vi "ScaleWaveData.vi"(8 "error in (no error)":errorcluster, 11 "dDataIn":dbl[](array[numeric])) -> (0 "error out":errorcluster, 3 "dDataOut":dbl[](array[numeric]))   [LabVIEW 2014, in "FGenPlugins.lvlib" / "NiPxi6733.lvclass"]
uses:
  NiPxi6733.lvclass
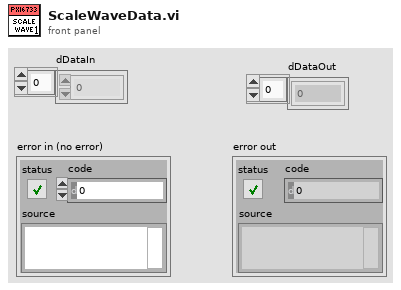
[diagram p1: front panel]
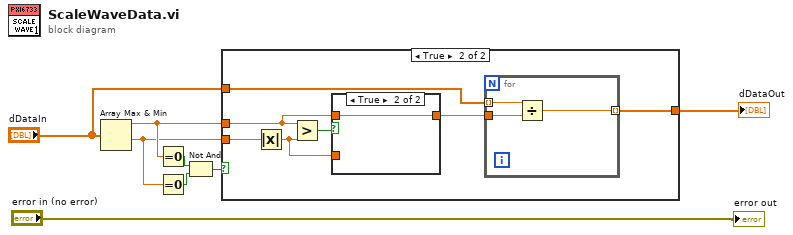
[diagram p0: block diagram]
diagram:
  n1 = Array Max & Min(array="dDataIn") -> (max value=w7:dbl, min value=w6:dbl)  [unwired: 2 out]
  n2 = Equal To 0?(x=w7) -> (x = 0?=w3:bool)
  n3 = Equal To 0?(x=w6) -> (x = 0?=w2:bool)
  n4 = Not And(1:w2, 2:w3) -> (0:w4:bool)
  n5 = case shown="True" w4 {
    tunnel: "dDataIn" -> [w9 w14]
    tunnel: w7 -> [_ w13]
    tunnel: w6 -> [_ w12]
    tunnel: [w9 w10] -> w5
    frame False {
    }
    frame True {
      n6 = Absolute Value(x=w12) -> (abs(x)=w15:dbl)
      n7 = Greater?(x=w13, y=w15) -> (0:w16:bool)
      n8 = case shown="True" w16 {
        tunnel: w13 -> [_ w21]
        tunnel: [w20 w21] -> w11
        tunnel: w15 -> [w20 _]
        frame False {
        }
        frame True {
        }
      }
      n9 = for {
        tunnel: w14 -> [w19] mode=indexing
        tunnel: w11 -> [w18]
        tunnel: [w17] -> w10 mode=indexing
        n10 = Divide(x=w19, y=w18) -> (x/y=w17:dbl)
      }
    }
  }
  "dDataOut" <- w5
  "error out" <- "error in (no error)"
